vi "Update VI in Library.vi"(8 "error in":errorcluster, 10 "VI":refnum<class "VI.lvclass">, 11 "Library in":refnum<class "Library.lvclass">) -> (0 "error out":errorcluster, 3 "Library out":refnum<class "Library.lvclass">)   [LabVIEW 2020, in "Panther Dashboard.lvlib" / "Library.lvclass"]
uses:
  Library.lvclass
  VI/VI.lvclass
  C:/GitClones/PantherDashboard/src/LabVIEW/Panther Dashboard/Class/LabVIEWItem/LabVIEWItem.lvclass
  Library.lvclass/Library.ctl
  LabVIEWItem/LabVIEWItem.lvclass/LabVIEWItem.ctl
  LabVIEWItem/Read Item Path.vi
  LabVIEWItem/Read Item Type.vi
  Read VIs MAP.vi
  Write VIs MAP.vi
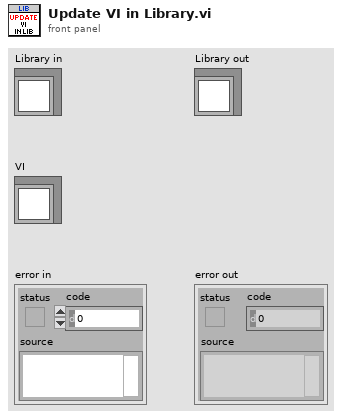
[diagram p1: front panel]
types:
  T1 = typedef "Panther Dashboard.lvlib/LabVIEWItem.lvclass/Item Type--enum.ctl" = enum16{"Requests", "Broadcasts", "Request and Wait for Reply", "Round Trip", "» Public API VIs", "» Constant VIs", "» Error VIs", "Module", "Project", "No Drag Selection"}
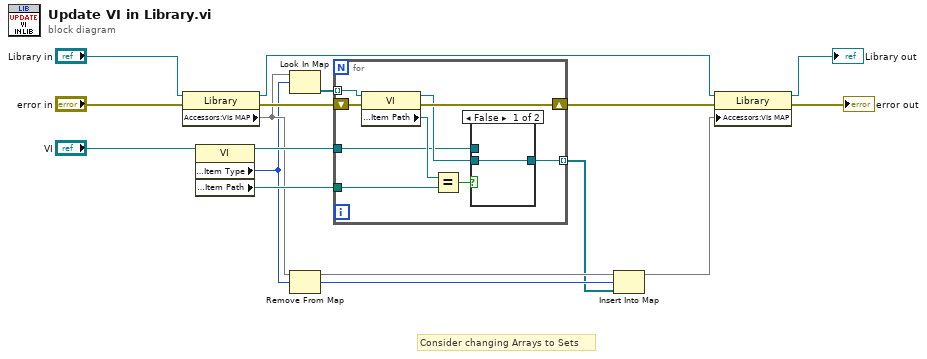
[diagram p0: block diagram]
diagram:
  # "Consider changing Arrays to Sets"
  n1 = property class="Library"(reference="Library in", error in="error in") -> (reference out=w11:refnum<class "Library.lvclass">, error out=w14:errorcluster, "Accessors:VIs MAP"=w5:map{T1, refnum<class "VI.lvclass">[]})
  n2 = property class="VI"(reference="VI") -> (reference out=w6:refnum<class "VI.lvclass">, "Accessors:Item Type"=w3:T1, "Accessors:Item Path"=w7:path)  [unwired: 1 in, 1 out]
  n3 = Look In Map(map=w5, key=w3) -> (value=w9:refnum<class "VI.lvclass">[])  [unwired: 1 in, 1 out]
  n4 = Remove From Map(10:w3, 11:w5) -> (3:w4:map{T1, refnum<class "VI.lvclass">[]})  [unwired: 2 out]
  n5 = for {
    tunnel: w9 -> [w23] mode=indexing
    tunnel: w7 -> [w21]
    tunnel: w6 -> [w17]
    tunnel: [w18] -> w2 mode=indexing
    shift-right: [w24] -> w13
    shift-left: w14 -> [w25]
    n6 = property class="VI"(reference=w23, error in=w25) -> (reference out=w19:refnum<class "VI.lvclass">, error out=w24:errorcluster, "Accessors:Item Path"=w22:path)
    n7 = Equal?(x=w22, y=w21) -> (x = y?=w20:bool)
    n8 = case shown="False" w20 {
      tunnel: [w26 w27] -> w18
      tunnel: w19 -> [w26 _]
      tunnel: w17 -> [_ w27]
      frame False {
      }
      frame True {
      }
    }
  }
  n9 = Insert Into Map(map in=w4, key=w3, value=w2) -> (map out=w1:map{T1, refnum<class "VI.lvclass">[]})  [unwired: 2 out]
  n10 = property class="Library"(reference=w11, error in=w13, "Accessors:VIs MAP"=w1) -> (reference out=→"Library out":refnum<class "Library.lvclass">, error out=→"error out":errorcluster)
